vi "Get Digital Input.vi"(9 "Use in Simulator (F)":bool, 11 "DigitalInput Refnum":string) -> (1 "Value":bool=TRUE)   [LabVIEW 2012]
uses:
  Robot Global Data.vi
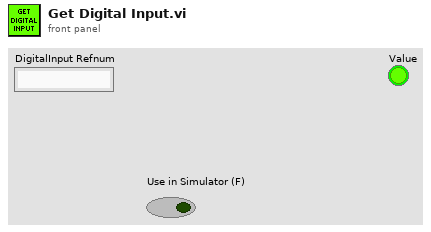
[diagram p1: front panel]
types:
  T1 = typedef "WPI_DigitalInputDevRef.ctl" = cluster{"DevStatus":errorcluster, "DIO Channel":T2, "Digital Module":T3}
  T2 = typedef "FPGA_DIOChannel.ctl" = enum8{"DIO 1", "DIO 2", "DIO 3", "DIO 4", "DIO 5", "DIO 6", "DIO 7", "DIO 8", "DIO 9", "DIO 10", "DIO 11", "DIO 12", "DIO 13", "DIO 14", "Invalid"}
  T3 = typedef "FPGA_TypedefDigitalModule.ctl" = enum16{"Digital Module 1", "Digital Module 2"}
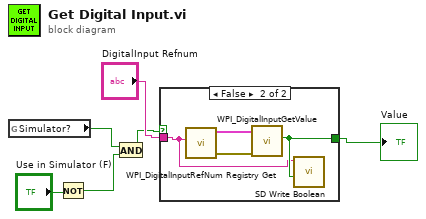
[diagram p0: block diagram]
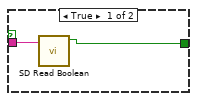
[diagram p2: hidden frame]
diagram:
  n1 = global read "Robot Global Data.vi" "Simulator?"() -> (w3:bool)
  n2 = Not(x="Use in Simulator (F)") -> (.not. x?=w2:bool)
  n3 = And(x=w3, y=w2) -> (x .and. y?=w1:bool)
  n4 = case shown="False" w1 {
    tunnel: "DigitalInput Refnum" -> [w7 w9]
    tunnel: [w8 w10] -> w5
    frame True {
      n5 = call <vilib>:"SD Read Boolean.vi"("Name"=w7) -> ("Boolean"=w8:bool)  [unwired: 8 in, 2 out]
    }
    frame False {
      n6 = call <vilib>:"WPI_DigitalInputRefNum Registry Get.vi"("refnum name"=w9) -> ("error out"=w11:errorcluster, "DigitalInputDevRef"=w12:T1)  [unwired: 9 in]
      n7 = call <vilib>:"WPI_DigitalInputGetValue.vi"("error in (no error)"=w11, "DigitalInputDevRef"=w12) -> ("Value"=w10:bool)  [unwired: 7 in, 2 out]
      n8 = call <vilib>:"SD Write Boolean.vi"("Boolean"=w10, "Name"=w9) -> ()  [unwired: 8 in, 2 out]
    }
  }
  "Value" <- w5
